vi "Command_Left_Joints.vi"(4 "Mode":enum32{"Position", "Velocity", "Effort"}(ring), 5 "node":string, 6 "error in":errorcluster, 9 "Goal":T1={"Label"="", "Arm Angles (degrees)"=[0.0, 0.0, 0.0, 0.0, 0.0, 0.0, 0.0]}) -> (0 "error out":errorcluster, 3 "JointCommand":T2={"Mode"=enum."Position", "Arm Angles"=[-0.7853981633974483, -0.7853981633974483, 0.0, 0.7853981633974483, 0.0, 1.5707963267948966, 0.0], "Angle Names"=["left_s0", "left_s1", "left_e0", "left_e1", "left_w0", "left_w1", "left_w2"]} {"Arm Angles" format="%.3f"})   [LabVIEW 2013]
uses:
  ROS/RosMessages/Clusters/JointCommand.ctl
  Arm Globals.vi
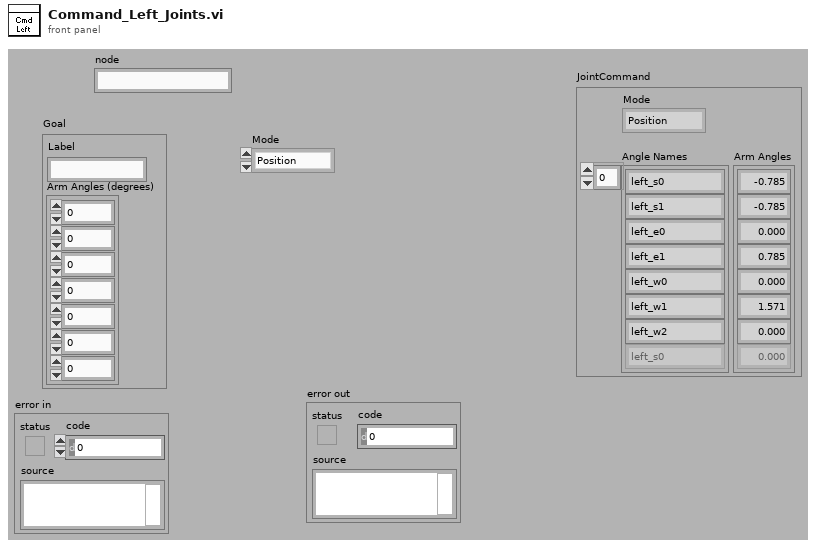
[diagram p1: front panel]
types:
  T1 = cluster{"Label":string, "Arm Angles (degrees)":dbl[]}
  T2 = typedef "JointCommand.ctl" = cluster{"Mode":enum32{"", "Position", "Velocity", "Effort"}, "Arm Angles":dbl[], "Angle Names":string[]}
  T3 = enum16{"big-endian, network order", "native, host order", "little-endian"}
  T4 = typedef "_ROSControl.ctl" = cluster{"topic port":u16, "Node":string, "topic":string, "type":string, "node port":u32, "error ":errorcluster, "Direction":T5, "APIs":string[]}
  T5 = typedef "_ROSDirection.ctl" = enum16{"Node", "Publisher", "Subscriber", "Service Client"}
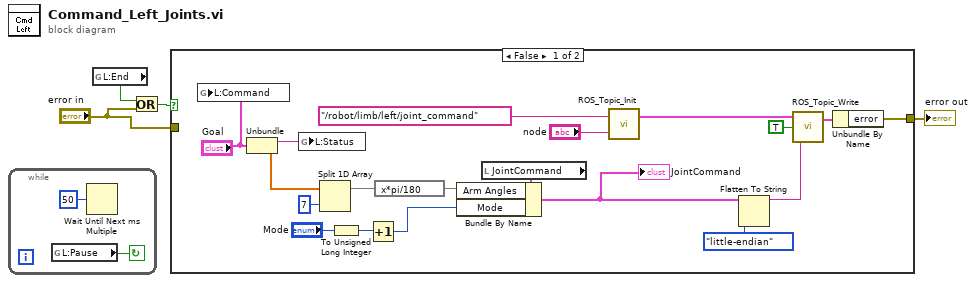
[diagram p0: block diagram]
diagram:
  n1 = while {
    stop <- w6 continue-if-true
    n2 = global read "Arm Globals.vi" "L:Pause"() -> (w6:bool)
    n3 = Wait Until Next ms Multiple(millisecond multiple=u32 50) -> ()  [unwired: 1 out]
  }
  n4 = global read "Arm Globals.vi" "L:End"() -> (w3:bool)
  n5 = Or(x=w3, y="error in") -> (x .or. y?=w2:bool)
  n6 = case shown="False" w2 {
    tunnel: [w25 w26] -> w4
    tunnel: "error in" -> [_ w26]
    frame False {
      n7 = global write "Arm Globals.vi" "L:Command"("Goal") -> ()
      n8 = Unbundle("Goal") -> ("Label"=w7:string, "Arm Angles (degrees)"=w9:dbl[])
      n9 = global write "Arm Globals.vi" "L:Status"(w7) -> ()
      n10 = Split 1D Array(array=w9, index=7) -> (first subarray=w11:dbl[])  [unwired: 1 out]
      n11 = To Unsigned Long Integer(number="Mode") -> (unsigned 32bit integer=w13:u32)
      n12 = Increment(x=w13) -> (x+1=w15:u32)
      n13 = expression code="x*pi/180"(w11) -> (w14:dbl[])
      n14 = local read "JointCommand"() -> (w12:T2)
      n15 = Bundle By Name(cluster=w12, "Arm Angles"=w14, "Mode"=w15) -> (w16:T2)
      "JointCommand" <- w16
      n16 = call "ROS_Topic_Init.vi"("node"="node", "topic"="/robot/limb/left/joint_command") -> ("ROS out"=w20:T4)  [unwired: 1 in]
      n17 = Flatten To String(anything=w16, byte order (0:big-endian, network order)=T3."little-endian") -> (data string=w23:string)  [unwired: 2 in, 2 out]
      n18 = call "ROS_Topic_Write.vi"("Msg in"=w23, "Continuous?"=TRUE, "ROS in"=w20) -> ("ROS out"=w19:T4)  [unwired: 1 in]
      n19 = Unbundle By Name(w19) -> ("error"=w25:errorcluster)
    }
    frame True {
    }
  }
  "error out" <- w4
